vi "Prüfstand.vi"() -> ()   [LabVIEW 2021]
uses:
  typedef/Main_Tabcontrol.ctl
  typedef/Channel_Information_Control_array.ctl
  typedef/Channel_Information_Control_single.ctl
  typedef/Sampling_Cluster.ctl
  typedef/Queue_Cluster.ctl
  <vilib>/DAQmx/read.llb/DAQmx Read (Analog 1D Wfm NChan NSamp).vi
  <vilib>/DAQmx/configure/timing.llb/DAQmx Timing (Sample Clock).vi
  <vilib>/DAQmx/configure/task.llb/DAQmx Configure Logging (TDMS).vi
  <vilib>/DAQmx/miscellaneous.llb/DAQmx Fill In Error Info.vi
panel:
  in  "Exit":bool
  in  "Main Control":T1
  in  "Load_Config":bool
  in  "Save_Config":bool
  in  "Verify_Channel_Settings":bool
  in  "Channel_Information_Control":T2 {"Input Terminal Configuration" items=["default"=-1, "RSE"=10083, "NRSE"=10078, "Differential"=10106, "Pseudodifferential"=12529]}
  in  "Drehzahl /min":dbl
  in  "Confirm_Save_File":bool
  in  "Add_Q_H_to_Graph":bool
  in  "Delete_Point":bool
  out "Current Measurement Values":waveform(dbl)[](graph)
  out "H-Q-Kennlinie":cluster{dbl[], dbl[]}(graph)
  in  "Cluster_Measurement":T4
  in  "Sampling_Information":T5={"sample mode"=10123, "Sample Rate (Hz)"=1000.0, "samples per channel"=1000} {"Sample Rate (Hz)" format="%#_13g"; "sample mode" items=["Finite Samples"=10178, "Continuous Samples"=10123, "Hardware Timed Single Point"=12522]}
  in  "Measurement file":path
  in  "Settings_H-Q-Kennlinie":T6
  out "error out":errorcluster
  # "not implemented correctly yet"
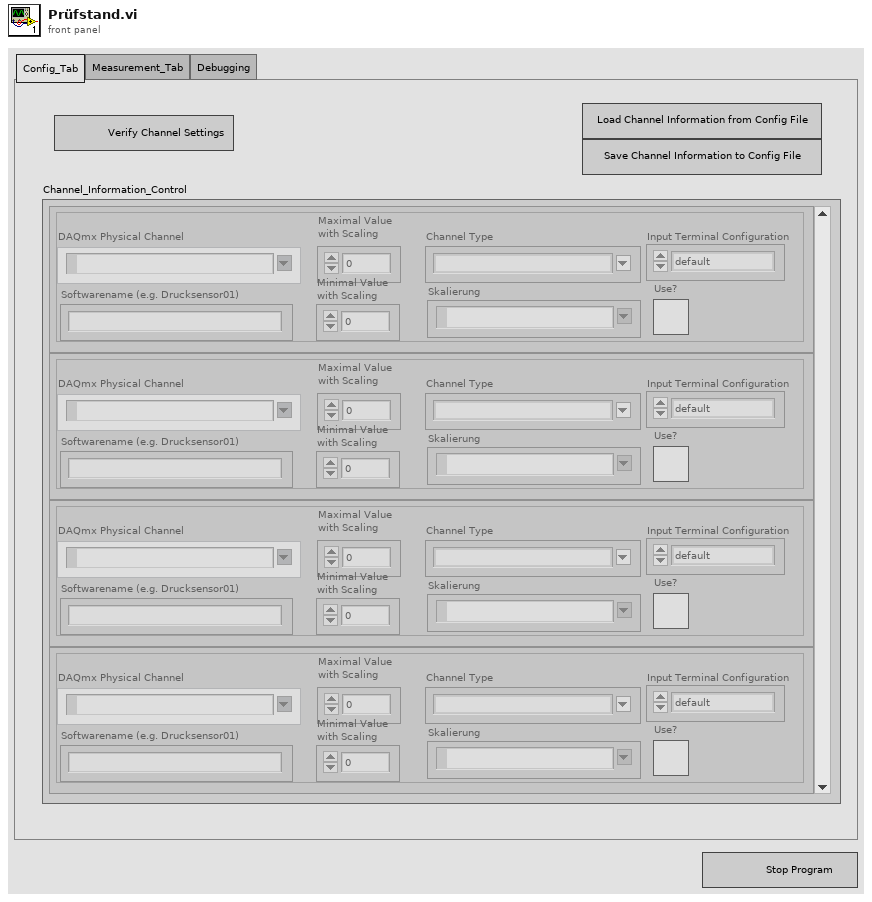
[diagram p1: front panel]
types:
  T1 = typedef "Main_Tabcontrol.ctl" = enum32{"Config_Tab", "Measurement_Tab", "Debugging"}
  T2 = typedef "Channel_Information_Control_array.ctl" = T3[]
  T3 = typedef "Channel_Information_Control_single.ctl" = cluster{"DAQmx Physical Channel":tag, "Softwarename (e.g. Drucksensor01)":string, "Maximal Value \nwith Scaling":dbl, "Minimal Value\nwith Scaling":dbl, "Channel Type":string, "Input Terminal Configuration":i32, "Skalierung":tag, "Use?":bool}
  T4 = cluster{"Start_Meas":bool, "Stop Button":bool, "TDMS_File_Viewer":bool}
  T5 = typedef "Sampling_Cluster.ctl" = cluster{"sample mode":i32, "Sample Rate (Hz)":dbl, "samples per channel":i32}
  T6 = cluster{"Index MID":dbl, "Index Drucksensor druckseitig":dbl, "Index Drucksensor saugseitig":dbl}
  T7 = typedef "Queue_Cluster.ctl" = cluster{"cmd":string, "Data":variant}
  T8 = enum32{"Page Enabled", "Page Disabled", "Page Disabled & Grayed"}
  T9 = enum8{"Enabled", "Disabled", "Disabled and Grayed Out"}
  T10 = cluster{"Main Control":T1, "Page Enabled State":enum32{"Page Enabled", "Page Disabled", "Page Disabled & Grayed"}}
  T11 = enum16{"open", "open or create", "create or replace", "create", "open (read-only)"}
  T12 = cluster{"Default_meas_path":path, "Selected_meas_file":path, "Default_Config":path}
  T13 = cluster{"Meas_running":bool, "Task_verified":bool, "Channel_Testing":bool}
  T14 = cluster{"Measurement_Data":waveform(dbl)[], "Flags":cluster{"Meas_running":bool, "Task_verified":bool, "Channel_Testing":bool}, "Channel_Information":T2, "Analog_Task":refnum<k21>, "Sampling_Information":T5, "Paths":cluster{"Default_meas_path":path, "Selected_meas_file":path, "Default_Config":path}}
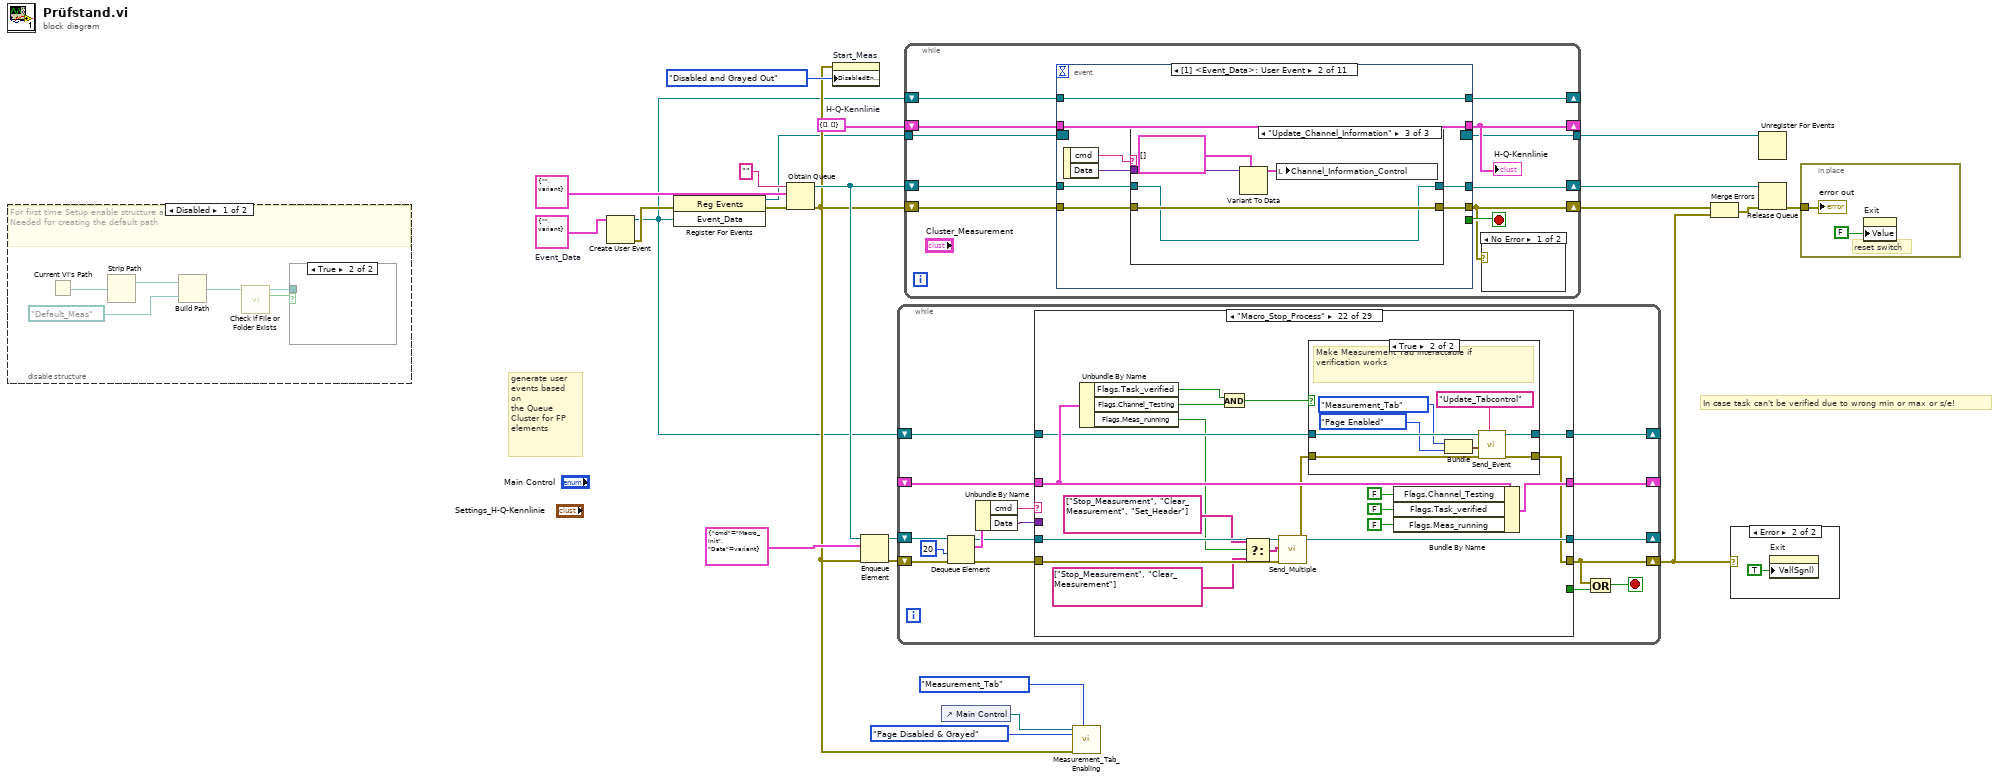
[diagram p0: block diagram]
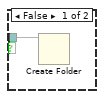
[diagram p2: hidden frame]
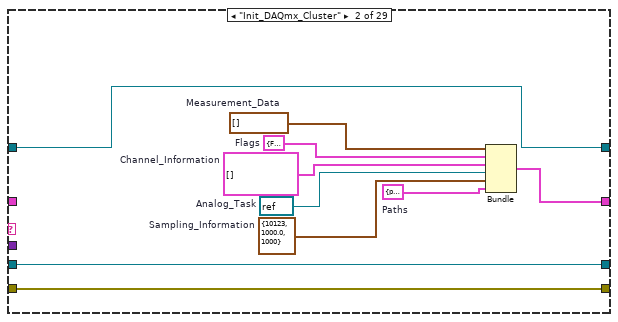
[diagram p6: hidden frame]
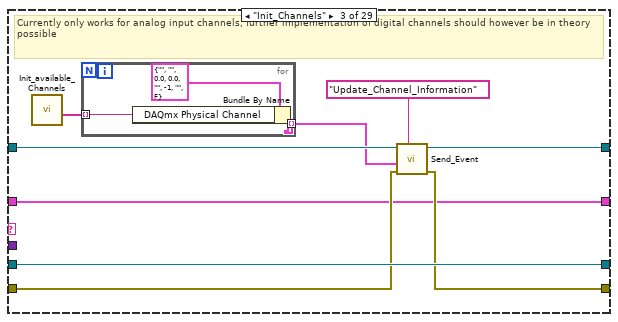
[diagram p7: hidden frame]
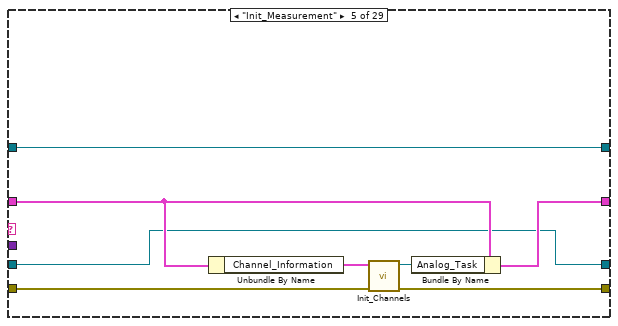
[diagram p9: hidden frame]
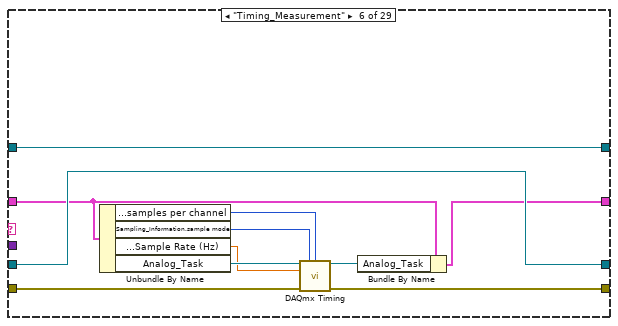
[diagram p10: hidden frame]
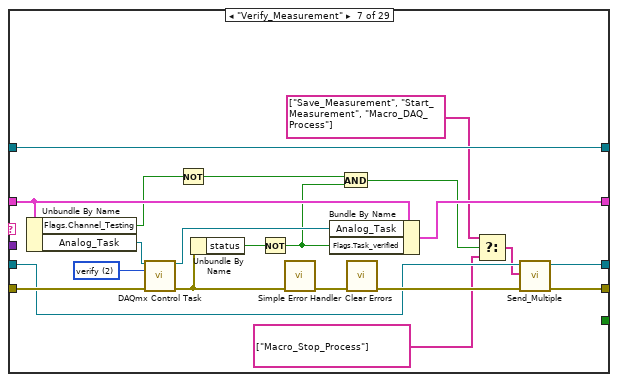
[diagram p11: hidden frame]
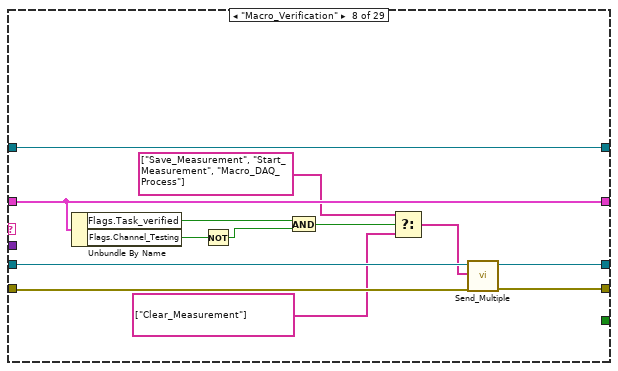
[diagram p12: hidden frame]
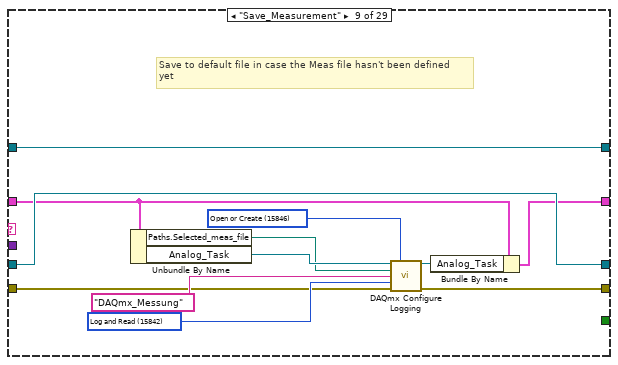
[diagram p13: hidden frame]
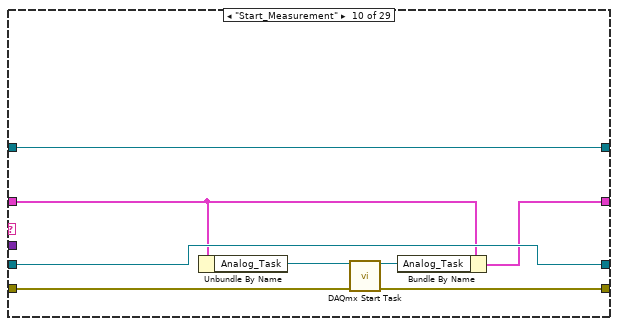
[diagram p14: hidden frame]
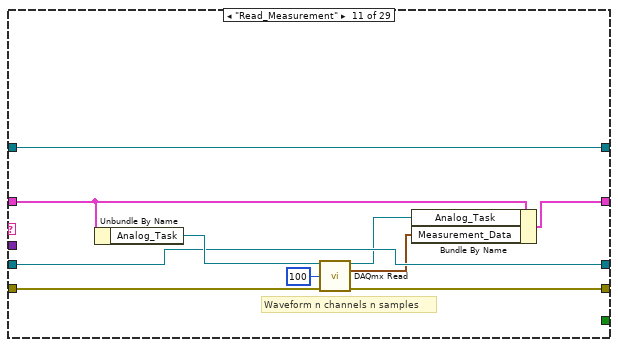
[diagram p15: hidden frame]
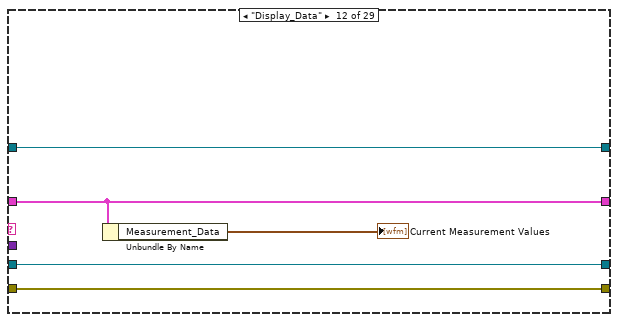
[diagram p16: hidden frame]
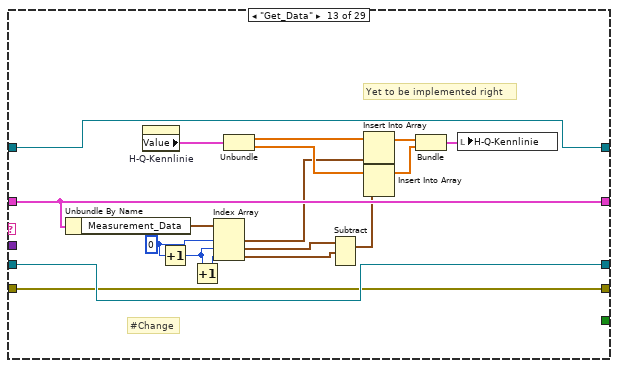
[diagram p17: hidden frame]
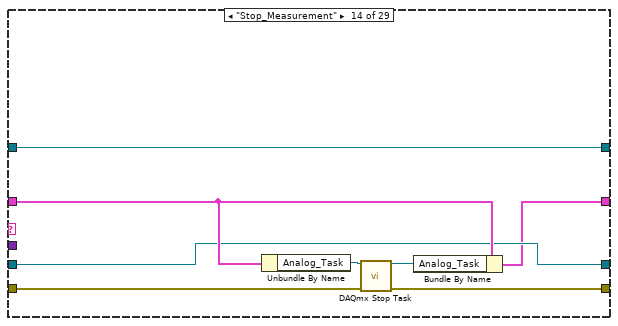
[diagram p18: hidden frame]
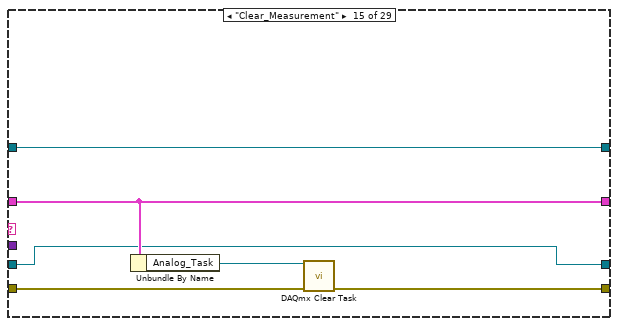
[diagram p19: hidden frame]
diagram:
  w1 = T7 {"cmd"="", "Data"=variant}  # Event_Data
  w19 = cluster{"Q/m³/h":dbl[], "H/m":dbl[]} {"Q/m³/h"=[], "H/m"=[]}  # H-Q-Kennlinie
  # "generate user events based on\nthe Queue Cluster for FP elements"
  # "In case task can't be verified due to wrong min or max or s/e!"
  n1 = disable-structure shown="Disabled" {
    frame Disabled {
      # "For first time Setup enable structure and run code!\nNeeded for creating the default path"
      n2 = Current VI's Path() -> (path=w29:path)
      n3 = Strip Path(path=w29) -> (stripped path=w28:path)  [unwired: 1 out]
      n4 = Build Path(base path=w28, name or relative path=path "Default_Meas") -> (appended path=w26:path)
      n5 = call <vilib>:"Check if File or Folder Exists.vi"("path"=w26) -> ("file or folder exists?"=w24:bool, "dup path"=w25:path)  [unwired: 8 in, 1 out]
      n6 = case shown="True" w24 {
        tunnel: w25 -> [w30 _]
        frame False {
          n7 = Create Folder(path (use dialog)=w30) -> ()  [unwired: 2 in, 3 out]
        }
        frame True {
        }
      }
    }
    frame Enabled {
    }
  }
  n8 = Create User Event(user event datatype=w1) -> (user event=w2:refnum<user-event>, error out=w7:errorcluster)  [unwired: 1 in]
  n9 = register-events(error in=w7, w2) -> (reference out=w5:refnum<event-registration>, error out=w8:errorcluster)  [unwired: 1 in]
  n10 = Obtain Queue(name (unnamed)="", element data type=T7 {"cmd"="", "Data"=variant}, error in (no error)=w8) -> (queue out=w15:refnum<queue>, error out=w10:errorcluster)  [unwired: 2 in, 1 out]
  n11 = property on="Start_Meas" class="Bool"(error in=w10, "DisabledEnum"=T9."Disabled and Grayed Out" ("Disabled")) -> ()  [unwired: 1 in, 2 out]
  n12 = Enqueue Element(queue=w15, element=T7 {"cmd"="Macro_Init", "Data"=variant}, error in (no error)=w10) -> (queue out=w14:refnum<queue>, error out=w13:errorcluster)  [unwired: 1 in, 1 out]
  n13 = while {
    shift-right: [w35] -> w18
    shift-left: w13 -> [w46]
    shift-right: [w39] -> _
    shift-left: w14 -> [w45]
    shift-right: [w38] -> _
    shift-left: _ -> [w37]
    shift-right: [w31] -> _
    shift-left: w2 -> [w32]
    stop <- w33 stop-if-true
    n14 = Dequeue Element(queue=w45, timeout in ms (-1)=20, error in (no error)=w46) -> (queue out=w41:refnum<queue>, element=w43:T7, error out=w40:errorcluster)  [unwired: 1 out]
    n15 = Unbundle By Name(w43) -> ("cmd"=w42:string, "Data"=w36:variant)
    n16 = case shown="\"Macro_Stop_Process\"" w42 {
      selector: w42 -> [_ _ _ _ _ _ _ _ _ _ _ _ _ _ _ _ _ _ _ _ _ _ _ _ _ _ _ _ w341]
      tunnel: w41 -> [w48 w60 w69 w74 w77 w92 w105 w125 w141 w146 w156 w164 w182 w186 w192 w200 w205 w221 w234 w257 w264 w285 w299 w309 w317 w321 w334 w339 w345]
      tunnel: w40 -> [w49 w59 w66 w73 w83 w94 w115 w124 w132 w149 w158 w163 w181 w190 w194 w199 w204 w220 w242 w256 w265 w286 w298 w310 w316 w320 w328 w338 w346]
      tunnel: [w49 w59 w65 w73 w82 w93 w107 w126 w133 w147 w157 w163 w181 w189 w193 w199 w203 w219 w227 w255 w262 w273 w298 w310 w316 w320 w331 w338 w346] -> w35
      tunnel: [w48 w60 w69 w74 w77 w92 w106 w127 w141 w146 w156 w164 w182 w186 w192 w200 w202 w218 w234 w254 w263 w284 w299 w309 w317 w321 w334 w339 w345] -> w39
      tunnel: [_ _ _ _ _ _ _ _ _ _ _ _ _ _ _ _ _ _ _ _ _ _ _ _ _ _ _ TRUE _] -> w34
      tunnel: [w50 w53 w63 w76 w79 w89 w110 w128 w138 w144 w152 w162 w180 w184 w196 w198 w207 w213 w233 w252 w267 w282 w300 w306 w313 w319 w324 w336 w344] -> w38
      tunnel: w37 -> [w50 _ w63 w76 w81 w91 w112 w128 w139 w145 w155 w162 w180 w187 w196 w198 w207 w214 w237 w249 w267 w279 w300 w303 w315 w319 w324 w336 w344]
      tunnel: w36 -> [_ _ _ _ _ _ _ _ _ _ _ _ _ _ _ _ _ w216 w241 w250 _ _ _ w311 _ _ _ _ _]
      tunnel: w32 -> [w47 w51 w68 w75 w78 w85 w104 w129 w130 w142 w150 w160 w165 w183 w191 w197 w206 w208 w230 w244 w258 w274 w297 w301 w312 w318 w322 w335 w340]
      tunnel: [w47 w51 w67 w75 w78 w85 w104 w129 w130 w142 w150 w160 w165 w183 w191 w197 w206 w208 w229 w244 w258 w272 w297 w301 w312 w318 w322 w335 w340] -> w31
      frame "---Init---" {
      }
      frame "Init_DAQmx_Cluster" {
        w52 = T12 {"Default_meas_path"=path "", "Selected_meas_file"=path "", "Default_Config"=path ""}  # Paths
        w54 = T5 {"sample mode"=10123, "Sample Rate (Hz)"=1000.0, "samples per channel"=1000}  # Sampling_Information
        w55 = refnum<k21> refnum  # Analog_Task
        w56 = T2 []  # Channel_Information
        w57 = T13 {"Meas_running"=FALSE, "Task_verified"=FALSE, "Channel_Testing"=FALSE}  # Flags
        w58 = waveform(dbl)[] []  # Measurement_Data
        n17 = Bundle("Measurement_Data"=w58, "Flags"=w57, "Channel_Information"=w56, "Analog_Task"=w55, "Sampling_Information"=w54, "Paths"=w52) -> (w53:T14)  [unwired: 1 in]
      }
      frame "Init_Channels" {
        # "Currently only works for analog input channels, further implementation of digital channels should however be in theory possible"
        n18 = call "Init_available_Channels.vi"() -> ("AI.PhysicalChans"=w62:tag[])  [unwired: 11 in]
        n19 = for {
          tunnel: w62 -> [w71] mode=indexing
          tunnel: [w70] -> w61 mode=indexing
          n20 = Bundle By Name(cluster=T3 {"DAQmx Physical Channel"="", "Softwarename (e.g. Drucksensor01)"="", "Maximal Value \nwith Scaling"=0.0, "Minimal Value\nwith Scaling"=0.0, "Channel Type"="", "Input Terminal Configuration"=-1, "Skalierung"="", "Use?"=FALSE} ("Channel_Information"), "DAQmx Physical Channel"=w71) -> (w70:T3)
        }
        n21 = call "Send_Event.vi"("cmd"="Update_Channel_Information", "Error in"=w66, "Data"=w61, "User Event in"=w68) -> ("error out"=w65:errorcluster, "User Event out"=w67:refnum<user-event>)  [unwired: 6 in]
      }
      frame "---Meas_Procedure---" {
      }
      frame "Init_Measurement" {
        n22 = Unbundle By Name(w81) -> ("Channel_Information"=w84:T2)
        n23 = call "Init_Channels.vi"("Error in"=w83, "Channel_Information"=w84) -> ("Error Out"=w82:errorcluster, "Task out"=w80:refnum<k21>)  [unwired: 8 in]
        n24 = Bundle By Name(cluster=w81, "Analog_Task"=w80) -> (w79:T14)
      }
      frame "Timing_Measurement" {
        n25 = Unbundle By Name(w91) -> ("Sampling_Information.samples per channel"=w88:i32, "Sampling_Information.sample mode"=w87:i32, "Sampling_Information.Sample Rate (Hz)"=w86:dbl, "Analog_Task"=w95:refnum<k21>)
        n26 = call-poly <vilib>:"DAQmx Timing.vi"("task/channels in"=w95, "sample mode"=w87, "samples per channel"=w88, "rate"=w86, "error in"=w94) -> ("task out"=w90:refnum<k21>, "error out"=w93:errorcluster)  [unwired: 9 in]
        n27 = Bundle By Name(cluster=w91, "Analog_Task"=w90) -> (w89:T14)
      }
      frame "Verify_Measurement" {
        w116 = 2 items=["verify"=2, "reserve"=4, "commit"=3, "unreserve"=5, "abort"=6] ("action")
        n28 = Unbundle By Name(w112) -> ("Flags.Channel_Testing"=w99:bool, "Analog_Task"=w113:refnum<k21>)
        n29 = call <vilib>:"DAQmx Control Task.vi"("task/channels in"=w113, "action"=w116, "error in"=w115) -> ("task out"=w111:refnum<k21>, "error out"=w109:errorcluster)  [unwired: 11 in]
        n30 = Not(x=w99) -> (.not. x?=w100:bool)
        n31 = Unbundle By Name(w109) -> ("status"=w96:bool)
        n32 = Not(x=w96) -> (.not. x?=w97:bool)
        n33 = call <vilib>:"Simple Error Handler.vi"("error in (no error)"=w109) -> ("error out"=w114:errorcluster)  [unwired: 4 in, 4 out]
        n34 = Bundle By Name(cluster=w112, "Analog_Task"=w111, "Flags.Task_verified"=w97) -> (w110:T14)
        n35 = And(x=w100, y=w97) -> (x .and. y?=w101:bool)
        n36 = call <vilib>:"Clear Errors.vi"("error in (no error)"=w114) -> ("error out"=w108:errorcluster)  [unwired: 5 in, 1 out]
        n37 = Select(t=string[] ["Save_Measurement", "Start_Measurement", "Macro_DAQ_Process"] ("Commands"), s=w101, f=string[] ["Macro_Stop_Process"]) -> (s? t:f=w102:string[])
        n38 = call "Send_Multiple.vi"("Error in"=w108, "Commands"=w102, "Queue_in"=w105) -> ("Error out"=w107:errorcluster, "Queue_out"=w106:refnum<queue>)  [unwired: 7 in]
      }
      frame "Macro_Verification" {
        n39 = Unbundle By Name(w128) -> ("Flags.Task_verified"=w122:bool, "Flags.Channel_Testing"=w121:bool)
        n40 = Not(x=w121) -> (.not. x?=w120:bool)
        n41 = And(x=w122, y=w120) -> (x .and. y?=w119:bool)
        n42 = Select(t=string[] ["Save_Measurement", "Start_Measurement", "Macro_DAQ_Process"] ("f"), s=w119, f=string[] ["Clear_Measurement"]) -> (s? t:f=w118:string[])
        n43 = call "Send_Multiple.vi"("Error in"=w124, "Commands"=w118, "Queue_in"=w125) -> ("Error out"=w126:errorcluster, "Queue_out"=w127:refnum<queue>)  [unwired: 7 in]
      }
      frame "Save_Measurement" {
        w135 = 15846 items=["Open"=10437, "Open or Create"=15846, "Create or Replace"=15847, "Create"=15848] ("operation")
        w136 = 15842 items=["Off"=10231, "Log"=15844, "Log and Read"=15842] ("logging mode")
        # "Save to default file in case the Meas file hasn't been defined\nyet"
        n44 = Unbundle By Name(w139) -> ("Paths.Selected_meas_file"=w131:path, "Analog_Task"=w140:refnum<k21>)
        n45 = call-poly <vilib>:"DAQmx Configure Logging.vi"("task/channels in"=w140, "operation"=w135, "file path"=w131, "group name"="DAQmx_Messung", "logging mode"=w136, "error in"=w132) -> ("task out"=w137:refnum<k21>, "error out"=w133:errorcluster)  [unwired: 8 in]
        n46 = Bundle By Name(cluster=w139, "Analog_Task"=w137) -> (w138:T14)
      }
      frame "Start_Measurement" {
        n47 = Unbundle By Name(w145) -> ("Analog_Task"=w148:refnum<k21>)
        n48 = call <vilib>:"DAQmx Start Task.vi"("task/channels in"=w148, "error in"=w149) -> ("task out"=w143:refnum<k21>, "error out"=w147:errorcluster)  [unwired: 12 in]
        n49 = Bundle By Name(cluster=w145, "Analog_Task"=w143) -> (w144:T14)
      }
      frame "Read_Measurement" {
        # "Waveform n channels n samples"
        n50 = Unbundle By Name(w155) -> ("Analog_Task"=w159:refnum<k21>)
        n51 = call-poly <vilib>:"DAQmx Read.vi"("task/channels in"=w159, "number of samples per channel"=100, "error in"=w158) -> ("task out"=w153:refnum<k21>, "data"=w154:waveform(dbl)[], "error out"=w157:errorcluster)  [unwired: 10 in]
        n52 = Bundle By Name(cluster=w155, "Analog_Task"=w153, "Measurement_Data"=w154) -> (w152:T14)
      }
      frame "Display_Data" {
        n53 = Unbundle By Name(w162) -> ("Measurement_Data"=→"Current Measurement Values":waveform(dbl)[])
      }
      frame "Get_Data" {
        w169 = 0 ("index")
        # "Yet to be implemented right"
        # "#Change"
        n54 = Unbundle By Name(w180) -> ("Measurement_Data"=w173:waveform(dbl)[])
        n55 = property on="H-Q-Kennlinie" class="XYGraph (strict)"() -> ("Value"=w179:cluster{dbl[], dbl[]})  [unwired: 2 in, 2 out]
        n56 = Increment(x=w169) -> (x+1=w168:i32)
        n57 = Increment(x=w168) -> (x+1=w167:i32)
        n58 = Index Array(array=w173, index #1=w169, index #2=w168, index #3=w167) -> (element #1=w172:waveform(dbl), element #2=w171:waveform(dbl), element #3=w170:waveform(dbl))
        n59 = Unbundle(w179) -> (w178:dbl[], w176:dbl[])
        n60 = Subtract(1:w170, 2:w171) -> (0:w166:waveform(dbl))  [unwired: 1 in, 1 out]
        n61 = Insert Into Array(array=w178, new element=w172) -> (w177:dbl[])  [unwired: 1 in]
        n62 = Insert Into Array(array=w176, new element=w166) -> (w175:dbl[])  [unwired: 1 in]
        n63 = Bundle(w177, w175) -> (w174:cluster{dbl[], dbl[]})  [unwired: 1 in]
        n64 = local write "H-Q-Kennlinie"(w174) -> ()
      }
      frame "Stop_Measurement" {
        n65 = Unbundle By Name(w187) -> ("Analog_Task"=w188:refnum<k21>)
        n66 = call <vilib>:"DAQmx Stop Task.vi"("task/channels in"=w188, "error in"=w190) -> ("task out"=w185:refnum<k21>, "error out"=w189:errorcluster)  [unwired: 12 in]
        n67 = Bundle By Name(cluster=w187, "Analog_Task"=w185) -> (w184:T14)
      }
      frame "Clear_Measurement" {
        n68 = Unbundle By Name(w196) -> ("Analog_Task"=w195:refnum<k21>)
        n69 = call <vilib>:"DAQmx Clear Task.vi"("task in"=w195, "error in"=w194) -> ("error out"=w193:errorcluster)  [unwired: 13 in]
      }
      frame "---Macros---" {
      }
      frame "Macro_Init" {
        n70 = call "Send_Multiple.vi"("Error in"=w204, "Commands"=string[] ["Init_DAQmx_Cluster", "Init_Channels"], "Queue_in"=w205) -> ("Error out"=w203:errorcluster, "Queue_out"=w202:refnum<queue>)  [unwired: 7 in]
      }
      frame "Macro_Init_Meas" {
        n71 = Unbundle By Name(w214) -> ("Sampling_Information"=w211:T5)
        n72 = Variant To Data(type=w211, Variant=w216) -> (data=w210:T5, error out=w215:errorcluster)  [unwired: 1 in]
        n73 = Select(t=w211, s=w215, f=w210) -> (s? t:f=w212:T5)
        n74 = call "Send_Multiple.vi"("Error in"=w220, "Commands"=string[] ["Init_Measurement", "Timing_Measurement", "Verify_Measurement"], "Queue_in"=w221) -> ("Error out"=w219:errorcluster, "Queue_out"=w218:refnum<queue>)  [unwired: 7 in]
        n75 = Bundle By Name(cluster=w214, "Flags.Meas_running"=TRUE, "Sampling_Information"=w212) -> (w213:T14)
      }
      frame "Macro_Load_Config" {
        n76 = Unbundle By Name(w237) -> ("Channel_Information"=w235:T2, "Paths.Default_Config"=w232:path)
        n77 = Variant To Data(type=w232, Variant=w241) -> (data=w239:path, error out=w240:errorcluster)  [unwired: 1 in]
        n78 = Select(t=w232, s=w240, f=w239) -> (s? t:f=w238:path)
        n79 = call "Load_Channel_Config_new.vi"("Error in"=w242, "configuration file path"=w238) -> ("Error out"=w228:errorcluster, "Channel_Information_Control"=w236:T2)  [unwired: 8 in]
        n80 = Select(t=w235, s=w228, f=w236) -> (s? t:f=w225:T2)
        n81 = To Variant(anything=w225) -> (Variant=w226:variant)
        n82 = To Variant(anything=T10 {"Main Control"=enum."Measurement_Tab", "Page Enabled State"=enum."Page Disabled & Grayed"} ("output cluster")) -> (Variant=w223:variant)
        n83 = Bundle By Name(cluster=w237, "Channel_Information"=w225) -> (w233:T14)
        n84 = Build Array(w226, w223) -> (w224:variant[])
        n85 = call "Send_Multiple_Event.vi"("cmd"=string[] ["Update_Channel_Information", "Update_Tabcontrol"], "Error in"=w228, "Data"=w224, "User Event in"=w230) -> ("Error out"=w227:errorcluster, "User Event"=w229:refnum<user-event>)  [unwired: 6 in]
      }
      frame "Macro_Test_Channels" {
        w251 = T5 {"sample mode"=10178, "Sample Rate (Hz)"=1000.0, "samples per channel"=100}  # Test_Sampling
        # "Test\nsample\nfor verification"
        n86 = Unbundle By Name(w249) -> ("Channel_Information"=w247:T2)
        n87 = Variant To Data(type=w247, Variant=w250) -> (data=w246:T2, error out=w248:errorcluster)  [unwired: 1 in]
        n88 = Select(t=w247, s=w248, f=w246) -> (s? t:f=w243:T2)
        n89 = call "Send_Multiple.vi"("Error in"=w256, "Commands"=string[] ["Init_Measurement", "Timing_Measurement", "Verify_Measurement"], "Queue_in"=w257) -> ("Error out"=w255:errorcluster, "Queue_out"=w254:refnum<queue>)  [unwired: 7 in]
        n90 = Bundle By Name(cluster=w249, "Sampling_Information"=w251, "Channel_Information"=w243, "Flags.Channel_Testing"=TRUE) -> (w252:T14)
      }
      frame "Macro_DAQ_Process" {
        n91 = Unbundle By Name(w267) -> ("Flags.Meas_running"=w266:bool)
        n92 = Select(t=string[] ["Read_Measurement", "Display_Data", "Macro_DAQ_Process"] ("Commands"), s=w266, f=string[] [""]) -> (s? t:f=w260:string[])
        n93 = call "Send_Multiple.vi"("Error in"=w265, "Commands"=w260, "Queue_in"=w264) -> ("Error out"=w262:errorcluster, "Queue_out"=w263:refnum<queue>)  [unwired: 7 in]
      }
      frame "Macro_Stop_Process" {
        n94 = Unbundle By Name(w279) -> ("Flags.Task_verified"=w271:bool, "Flags.Channel_Testing"=w270:bool, "Flags.Meas_running"=w268:bool)
        n95 = And(x=w271, y=w270) -> (x .and. y?=w269:bool)
        n96 = Select(t=string[] ["Stop_Measurement", "Clear_Measurement", "Set_Header"] ("Commands"), s=w268, f=string[] ["Stop_Measurement", "Clear_Measurement"] ("Commands")) -> (s? t:f=w278:string[])
        n97 = call "Send_Multiple.vi"("Error in"=w286, "Commands"=w278, "Queue_in"=w285) -> ("Error out"=w275:errorcluster, "Queue_out"=w284:refnum<queue>)  [unwired: 7 in]
        n98 = case shown="True" w269 {
          tunnel: w275 -> [w288 w294]
          tunnel: w274 -> [w287 w296]
          tunnel: [w288 w293] -> w273
          tunnel: [w287 w295] -> w272
          frame False {
          }
          frame True {
            # "Make Measurement Tab interactable if verification works"
            n99 = Bundle("Main Control"=Main_Tabcontrol."Measurement_Tab", "Page Enabled State"=T8."Page Enabled") -> (w289:T10)  [unwired: 1 in]
            n100 = call "Send_Event.vi"("cmd"="Update_Tabcontrol", "Error in"=w294, "Data"=w289, "User Event in"=w296) -> ("error out"=w293:errorcluster, "User Event out"=w295:refnum<user-event>)  [unwired: 6 in]
          }
        }
        n101 = Bundle By Name(cluster=w279, "Flags.Channel_Testing"=FALSE, "Flags.Task_verified"=FALSE, "Flags.Meas_running"=FALSE) -> (w282:T14)
      }
      frame "---GUI_Interaction---" {
      }
      frame "Update_Channel_Information" {
        w308 = T2 []  # Channel_Information_Control
        n102 = Variant To Data(type=w308, Variant=w311) -> (data=w304:T2, error out=w307:errorcluster)  [unwired: 1 in]
        n103 = Unbundle By Name(w303) -> ("Channel_Information"=w302:T2)
        n104 = Select(t=w302, s=w307, f=w304) -> (s? t:f=w305:T2)
        n105 = Bundle By Name(cluster=w303, "Channel_Information"=w305) -> (w306:T14)
      }
      frame "Update_Meas_File" {
        n106 = Bundle By Name(cluster=w315, "Paths.Selected_meas_file"="Measurement file") -> (w313:T14)
      }
      frame "" {
      }
      frame "Set_Header" {
        # "Set Header after the Task has been stopped"
        n107 = Unbundle By Name(w324) -> ("Paths.Selected_meas_file"=w323:path)
        n108 = TDMS Open(8:w328, 10:T11."open or create" ("operation (0:open)"), 11:w323) -> (0:w327:errorcluster, 3:w325:refnum<k34>)  [unwired: 4 in]
        n109 = TDMS Set Properties(5:"Drehzahl /min", 7:"Drehzahl", 8:w327, 11:w325) -> (0:w333:errorcluster, 3:w332:refnum<k34>)  [unwired: 2 in, 2 out]
        n110 = TDMS Close(8:w333, 11:w332) -> (0:w331:errorcluster)  [unwired: 1 out]
      }
      frame "Exit" {
      }
      frame Default {
        n111 = Concatenate Strings("Unknown Command:\n" ("string"), w341) -> (w343:string)
        n112 = One Button Dialog(message=w343) -> ()  [unwired: 1 in, 1 out]
      }
    }
    n113 = Compound Arithmetic op=OR(w35, w34) -> (w33:bool)
  }
  n114 = while {
    shift-right: [w354] -> w20
    shift-left: w15 -> [w356]
    shift-right: [w351] -> w22
    shift-left: w10 -> [w355]
    shift-right: [w352] -> _
    shift-left: w19 -> [w353]
    tunnel: w5 -> [w350]
    tunnel: [w349] -> w4
    shift-right: [w347] -> _
    shift-left: w2 -> [w348]
    stop <- w357 stop-if-true
    n115 = event shown="[1] <Event_Data>: User Event" {
      selector: w350 -> [_ _ _ _ _ _ _ _ _ _ _]
      dyn-events: [_ _ _ _ _ _ _ _ _ _ _] -> w349
      timeout: _ -> [_ _ _ _ _ _ _ _ _ _ _]
      tunnel: ["Exit" _ _ _ _ _ _ _ _ _ _] -> w357
      tunnel: w356 -> [w360 w371 w403 w410 w425 w438 w448 w455 w463 w476 w481]
      tunnel: w355 -> [w362 w375 w402 w412 w432 w437 w447 w456 w465 w475 w486]
      tunnel: [w364 w372 w402 w411 w419 w436 w446 w452 w461 w474 w482] -> w351
      tunnel: [w367 w370 w403 w410 w424 w435 w445 w453 w460 w473 w481] -> w354
      tunnel: w353 -> [w366 w374 w400 w409 w431 w439 w449 w457 w466 w477 w487]
      tunnel: [w366 w374 w396 w409 w431 w439 w449 w457 w466 w477 w487] -> w352
      tunnel: w348 -> [w359 w369 w394 w404 w417 w433 w440 w450 w458 w470 w485]
      tunnel: [w359 w369 w394 w404 w417 w433 w440 w450 w458 w470 w484] -> w347
      event "Exit": Value Change {
        # "Clear Error so\nthe Exit Command is sent\nto consumer"
        # "in case of errors till send the exit signal to consumer"
        n116 = event-data() -> ()  [unwired: 1 in, 2 out]
        n117 = call <vilib>:"Clear Errors.vi"("error in (no error)"=w362) -> ("error out"=w361:errorcluster)  [unwired: 5 in, 1 out]
        n118 = Enqueue Element(queue=w360, element=T7 {"cmd"="Exit", "Data"=variant}, error in (no error)=w361) -> (queue out=w367:refnum<queue>, error out=w365:errorcluster)  [unwired: 1 in, 1 out]
        n119 = Merge Errors(w365, w362) -> (w364:errorcluster)
      }
      event User Event {
        n120 = event-data() -> ("cmd"=w376:string, "Data"=w373:variant)  [unwired: 1 in]
        n121 = case shown="\"Update_Channel_Information\"" w376 {
          tunnel: w375 -> [w378 w386 w393]
          tunnel: w373 -> [_ w387 w392]
          tunnel: [w378 w384 w393] -> w372
          tunnel: w371 -> [w377 w383 w391]
          tunnel: [w377 w383 w391] -> w370
          frame Default {
          }
          frame "Update_Tabcontrol" {
            n122 = Variant To Data(error in=w386, type=T10 {"Main Control"=enum."Config_Tab", "Page Enabled State"=enum."Page Enabled"} ("output cluster"), Variant=w387) -> (data=w381:T10, error out=w385:errorcluster)
            n123 = Unbundle By Name(w381) -> ("Main Control"=w380:T1, "Page Enabled State"=w379:T8)
            n124 = control-ref of="Main Control"() -> (w388:refnum<vi>)
            n125 = call "Measurement_Tab_Enabling.vi"("Page_Label"=w380, "Error in"=w385, "Page_State"=w379, "TabControl in"=w388) -> ("Error out"=w384:errorcluster)  [unwired: 7 in]
          }
          frame "Update_Channel_Information" {
            n126 = Variant To Data(type=T2 [] ("s? t:f"), Variant=w392) -> (data=w389:T2)  [unwired: 1 in, 1 out]
            n127 = local write "Channel_Information_Control"(w389) -> ()
          }
        }
      }
      event "Delete_Point": Value Change {
        n128 = event-data() -> ()  [unwired: 1 in, 3 out]
        n129 = property on="H-Q-Kennlinie" class="XYGraph (strict)"() -> ("Cursor.Cursor Index"=w395:i32)  [unwired: 2 in, 2 out]
        n130 = Unbundle By Name(w400) -> ("Q/m³/h"=w401:dbl[], "H/m"=w397:dbl[])
        n131 = Delete From Array(array=w401, index=w395) -> (array with subset deleted=w399:dbl[])  [unwired: 1 in, 1 out]
        n132 = Delete From Array(array=w397, index=w395) -> (array with subset deleted=w398:dbl[])  [unwired: 1 in, 1 out]
        n133 = Bundle By Name(cluster=w400, "Q/m³/h"=w399, "H/m"=w398) -> (w396:cluster{"Q/m³/h":dbl[], "H/m":dbl[]})
      }
      event "Save_Config": Value Change {
        n134 = event-data() -> ()  [unwired: 1 in, 1 out]
        n135 = local read "Channel_Information_Control"() -> (w406:T2)
        n136 = call "File Dialog"("default name"="Default_Config", "error in"=w412, "pattern (all files)"="*.ini", "pattern label"=".ini") -> ("selected path"=w405:path, "error out"=w408:errorcluster)  [unwired: 8 in, 2 out]
        n137 = call "Save_Channel_Config.vi"("Error in"=w408, "configuration file path"=w405, "Channel_Information_Control"=w406) -> ("error out"=w407:errorcluster)  [unwired: 8 in]
        n138 = call <vilib>:"Clear Errors.vi"("error in (no error)"=w407, "specific error code to clear (0: all)"=43) -> ("error out"=w411:errorcluster)  [unwired: 4 in, 1 out]
      }
      event "Load_Config": Value Change {
        n139 = event-data() -> ()  [unwired: 1 in, 3 out]
        n140 = call "File Dialog2"("default name"="Default_Config", "error in"=w432, "pattern (all files)"="*.ini", "pattern label"=".ini") -> ("selected path"=w420:path, "error out"=w426:errorcluster)  [unwired: 8 in, 2 out]
        n141 = call <vilib>:"Clear Errors.vi"("error in (no error)"=w426, "specific error code to clear (0: all)"=43) -> ("error out"=w418:errorcluster)  [unwired: 4 in, 1 out]
        n142 = Bundle By Name(cluster=T7 {"cmd"="", "Data"=variant} ("element"), "cmd"="Macro_Load_Config", "Data"=w420) -> (w422:T7)
        n143 = Enqueue Element(queue=w425, element=w422, error in (no error)=w418) -> (queue out=w424:refnum<queue>, error out=w419:errorcluster)  [unwired: 1 in, 1 out]
      }
      event "Add_Q_H_to_Graph": Value Change {
        n144 = event-data() -> ()  [unwired: 1 in, 3 out]
        n145 = Enqueue Element(queue=w438, element=T7 {"cmd"="Get_Data", "Data"=variant}, error in (no error)=w437) -> (queue out=w435:refnum<queue>, error out=w436:errorcluster)  [unwired: 1 in, 1 out]
      }
      event "Cluster_Measurement.Start_Meas": Value Change {
        n146 = event-data() -> ()  [unwired: 1 in, 2 out]
        n147 = Bundle By Name(cluster=T7 {"cmd"="", "Data"=variant} ("element"), "cmd"="Macro_Init_Meas", "Data"="Sampling_Information") -> (w443:T7)
        n148 = Enqueue Element(queue=w448, element=w443, error in (no error)=w447) -> (queue out=w445:refnum<queue>, error out=w446:errorcluster)  [unwired: 1 in, 1 out]
      }
      event "Cluster_Measurement.Stop Button": Value Change {
        n149 = event-data() -> ()  [unwired: 1 in, 2 out]
        n150 = property on="Start_Meas" class="Bool"("DisabledEnum"=T9."Disabled and Grayed Out" ("Disabled")) -> ()  [unwired: 2 in, 2 out]
        n151 = Enqueue Element(queue=w455, element=T7 {"cmd"="Macro_Stop_Process", "Data"=variant}, error in (no error)=w456) -> (queue out=w453:refnum<queue>, error out=w452:errorcluster)  [unwired: 1 in, 1 out]
      }
      event "Confirm_Save_File": Value Change {
        n152 = event-data() -> ()  [unwired: 1 in, 2 out]
        n153 = property on="Start_Meas" class="Bool"(error in=w465, "DisabledEnum"=T9."Enabled" ("Disabled")) -> (error out=w462:errorcluster)  [unwired: 1 in, 1 out]
        n154 = Enqueue Element(queue=w463, element=T7 {"cmd"="Update_Meas_File", "Data"=variant}, error in (no error)=w462) -> (queue out=w460:refnum<queue>, error out=w461:errorcluster)  [unwired: 1 in, 1 out]
      }
      event "Verify_Channel_Settings": Value Change {
        n155 = event-data() -> ()  [unwired: 1 in, 2 out]
        n156 = call "Filter_Channel_Information.vi"("Channel_Information_Control"="Channel_Information_Control") -> ("Array"=w468:T3[])  [unwired: 10 in]
        n157 = Bundle By Name(cluster=T7 {"cmd"="", "Data"=variant} ("Queue_Cluster"), "cmd"="Macro_Test_Channels", "Data"=w468) -> (w472:T7)
        n158 = Enqueue Element(queue=w476, element=w472, error in (no error)=w475) -> (queue out=w473:refnum<queue>, error out=w474:errorcluster)  [unwired: 1 in, 1 out]
      }
      event Value Change {
        n159 = event-data() -> ()  [unwired: 1 in, 2 out]
        n160 = Bundle("Main Control"=Main_Tabcontrol."Measurement_Tab", "Page Enabled State"=T8."Page Disabled & Grayed") -> (w478:T10)  [unwired: 1 in]
        n161 = call "Send_Event.vi"("cmd"="Update_Tabcontrol", "Error in"=w486, "Data"=w478, "User Event in"=w485) -> ("error out"=w482:errorcluster, "User Event out"=w484:refnum<user-event>)  [unwired: 6 in]
      }
    }
    "H-Q-Kennlinie" <- w352
    n162 = case shown="No Error" w351 {
      frame No Error {
      }
      frame Error {
        n163 = property on="Exit" class="Bool (strict)"("Val(Sgnl)"=TRUE ("Value (Signaling)")) -> ()  [unwired: 2 in, 2 out]
      }
    }
  }
  n164 = control-ref of="Main Control"() -> (w11:refnum<vi>)
  n165 = call "Measurement_Tab_Enabling.vi"("Page_Label"=Main_Tabcontrol."Measurement_Tab" ("Main Control"), "Error in"=w10, "Page_State"=T8."Page Disabled & Grayed" ("Page Enabled State"), "TabControl in"=w11) -> ()  [unwired: 7 in, 1 out]
  n166 = Merge Errors(w22, w18) -> (w21:errorcluster)
  n167 = case shown="Error" w18 {
    frame No Error {
    }
    frame Error {
      n168 = property on="Exit" class="Bool (strict)"("Val(Sgnl)"=TRUE ("Value (Signaling)")) -> ()  [unwired: 2 in, 2 out]
    }
  }
  n169 = Unregister For Events(event registration refnum=w4) -> ()  [unwired: 1 in, 1 out]
  n170 = Release Queue(queue=w20, error in (no error)=w21) -> (error out=w17:errorcluster)  [unwired: 1 in, 2 out]
  n171 = in-place {
    in-place-border: w17 -> [w489]
    # "reset switch"
    n172 = property on="Exit" class="Bool (strict)"("Value"=FALSE ("Exit")) -> ()  [unwired: 2 in, 2 out]
    "error out" <- w489
  }
